vi "cryo v9.43.vi"() -> ()   [LabVIEW 2012]
uses:
  <vilib>/userdefined/High Color/IMAQdx.ctl
  <vilib>/Utility/file.llb/Read From Spreadsheet File (DBL).vi
  <vilib>/vision/driver/NI_Vision_Acquisition_Software.lvlib
  <vilib>/vision/NI_Vision_Development_Module.lvlib
panel:
  in  "Save\nImage":bool
  in  "Gap":u8=100
  in  "Position\nEstimate":dbl=20.0
  in  "Conn\nStm32":bool
  out "数值显示控件":dbl
  in  "停止按钮":bool
  in  "搜索按钮":bool
  out "Heater":u32(slide) scale=0.0..100.0
  out "数值 5":dbl
  out "数据显示 2":cluster{i32, dbl, dbl[][]}(graph)
  in  "文件路径输入控件 4":path=path "D:/testsizeout.txt"
  in  "多列列表框 3":i32(listbox)
  in  "Threshold Value":cluster{i32, i32}(slide)={180, 255} scale=0.0..255.0
  in  "文件路径输入控件 5":path=path "D:/testvideoin.avi"
  out "Source Image 5":T1(plugin-control) caption="Rejected Border"
  out "Source Image 4":T1(plugin-control) caption="Rejected Border"
  out "Source Image 3":T1(plugin-control) caption="Rejected Border"
  out "Source Image 2":T1(plugin-control) caption="Rejected Border"
  out "Source Image":T1(plugin-control) caption="Rejected Border"
  in  "Font, Size & Style":T2={"Desired Font (Application)"=enum."Application Font", "[User-specified Font]"={"Font Name"="", "Size"=12, "Strikeout?"=FALSE, "Italic?"=FALSE, "Underline?"=FALSE, "Outline?"=FALSE, "Shadow?"=FALSE, "Bold?"=FALSE, "Rotation Angle"=0.0}, "Horizontal Alignment"=0, "Vertical Alignment"=0} {"Vertical Alignment" items=["Bottom", "Top", "Baseline"]; "Horizontal Alignment" items=["Left", "Center", "Right"]; "[User-specified Font]"."Rotation Angle" format="%.2f"}
  in  "文件路径输入控件 3":path=path "D:/testvideoout.avi"
  in  "文件路径输入控件 2":path=path "D:/testprocessin.txt"
  in  "文件路径输入控件":path=path "D:/testtmpout.txt"
  in  "退出":bool
  in  "多列列表框 2":i32(listbox)
  in  "建立过程":bool
  in  "开始采集":bool
  out "数据显示":cluster{"x0":i32, "y":dbl, dbl[]}(graph)
  in  "停止采集":bool
  out "tmp":dbl(slide) scale=-50.0..50.0
  out "Injector 1":u32(slide) scale=0.0..100.0
  out "Injector 2":u32(slide) scale=0.0..100.0
  out "Injector 3":u32(slide) scale=0.0..100.0
  out "Refrigerator":u32(slide) scale=0.0..100.0
  out "数值 1":dbl
  out "数值 2":dbl
  out "数值 3":dbl
  out "数值 4":dbl
  out "多列列表框":i32[](listbox)
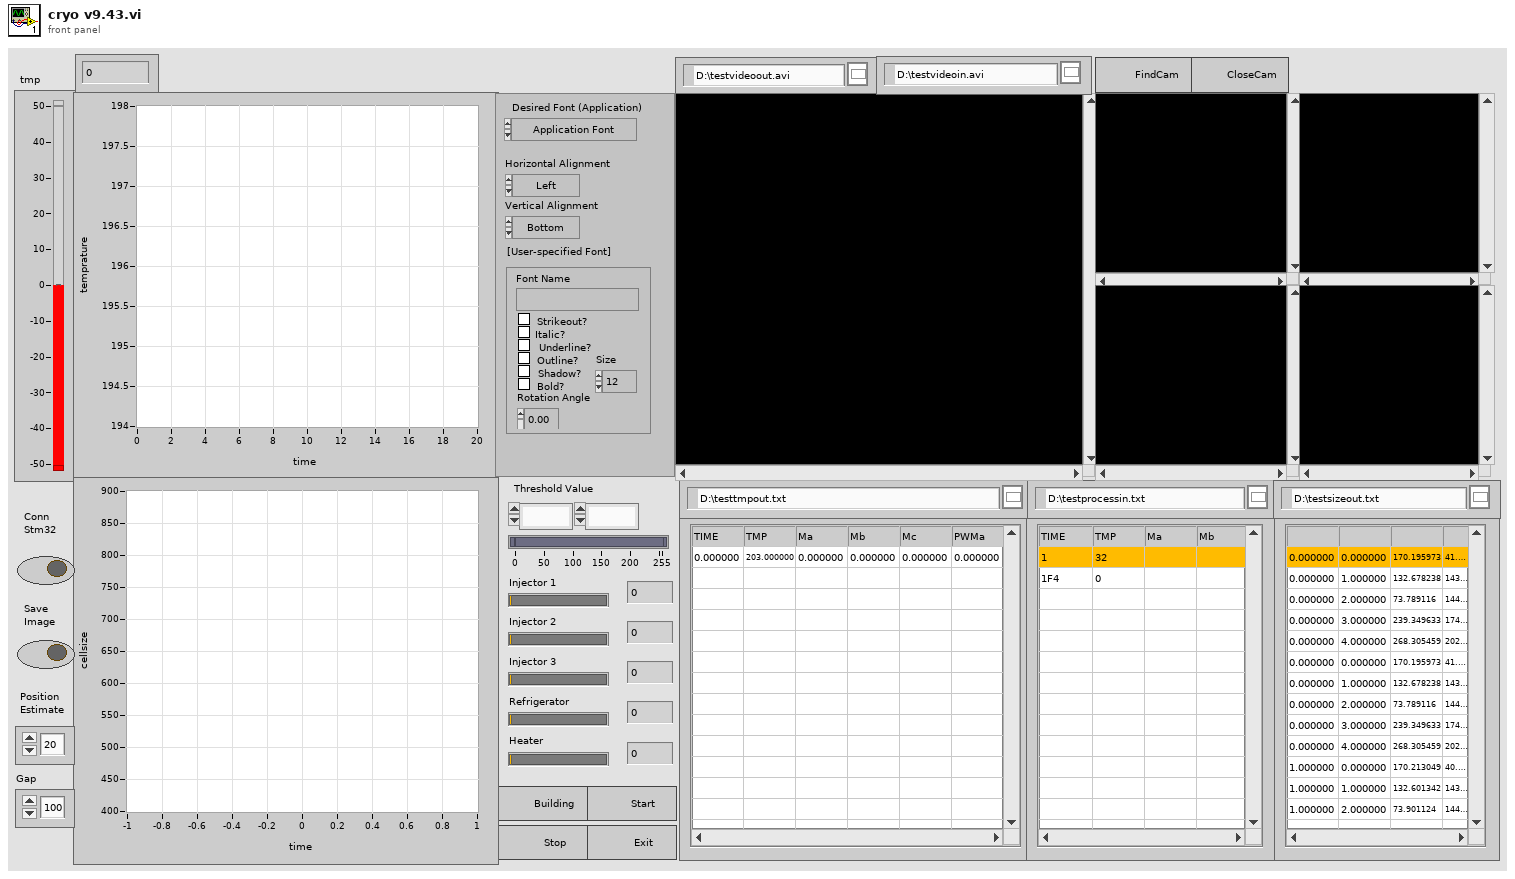
[diagram p1: front panel]
types:
  T1 = typedef "IMAQ Image.ctl" = refnum<image>
  T2 = cluster{"Desired Font (Application)":enum16{"User-specified Font", "Application Font", "System Font", "Dialog Font"}, "[User-specified Font]":cluster{"Font Name":string, "Size":i16, "Strikeout?":bool, "Italic?":bool, "Underline?":bool, "Outline?":bool, "Shadow?":bool, "Bold?":bool, "Rotation Angle":dbl}, "Horizontal Alignment":i16, "Vertical Alignment":i16}
  T3 = typedef "AviRefnum.ctl" = refnum<k1>
  T4 = typedef "Particle Parameters" = i32
  T5 = cluster{"Measurement Parameter":T4, "Range Lower Value":dbl, "Range Upper Value":dbl, "Range":bool, "Measurement Type":bool}[]
  T6 = enum32{"", "Gradient", "Laplacian", "Smoothing", "Gaussian"}
  T7 = cluster{"Particle Measurements (Pixels)[0]":dbl, "Particle Measurements (Pixels)[1]":dbl, "Particle Measurements (Pixels)[2]":dbl}
  T8 = cluster{"Particle Measurements (Pixels)[0]":dbl, "Particle Measurements (Pixels)[1]":dbl}
  T9 = cluster{i32, "Particle Measurements (Pixels)[0]":dbl, "Particle Measurements (Pixels)[1]":dbl, "Particle Measurements (Pixels)[2]":dbl, i32}
  T10 = cluster{i32, "Particle Measurements (Pixels)[0]":dbl, "Particle Measurements (Pixels)[1]":dbl, "Particle Measurements (Pixels)[2]":dbl, i32}[]
  T11 = typedef "IMAQdx.ctl" = refnum<k21>
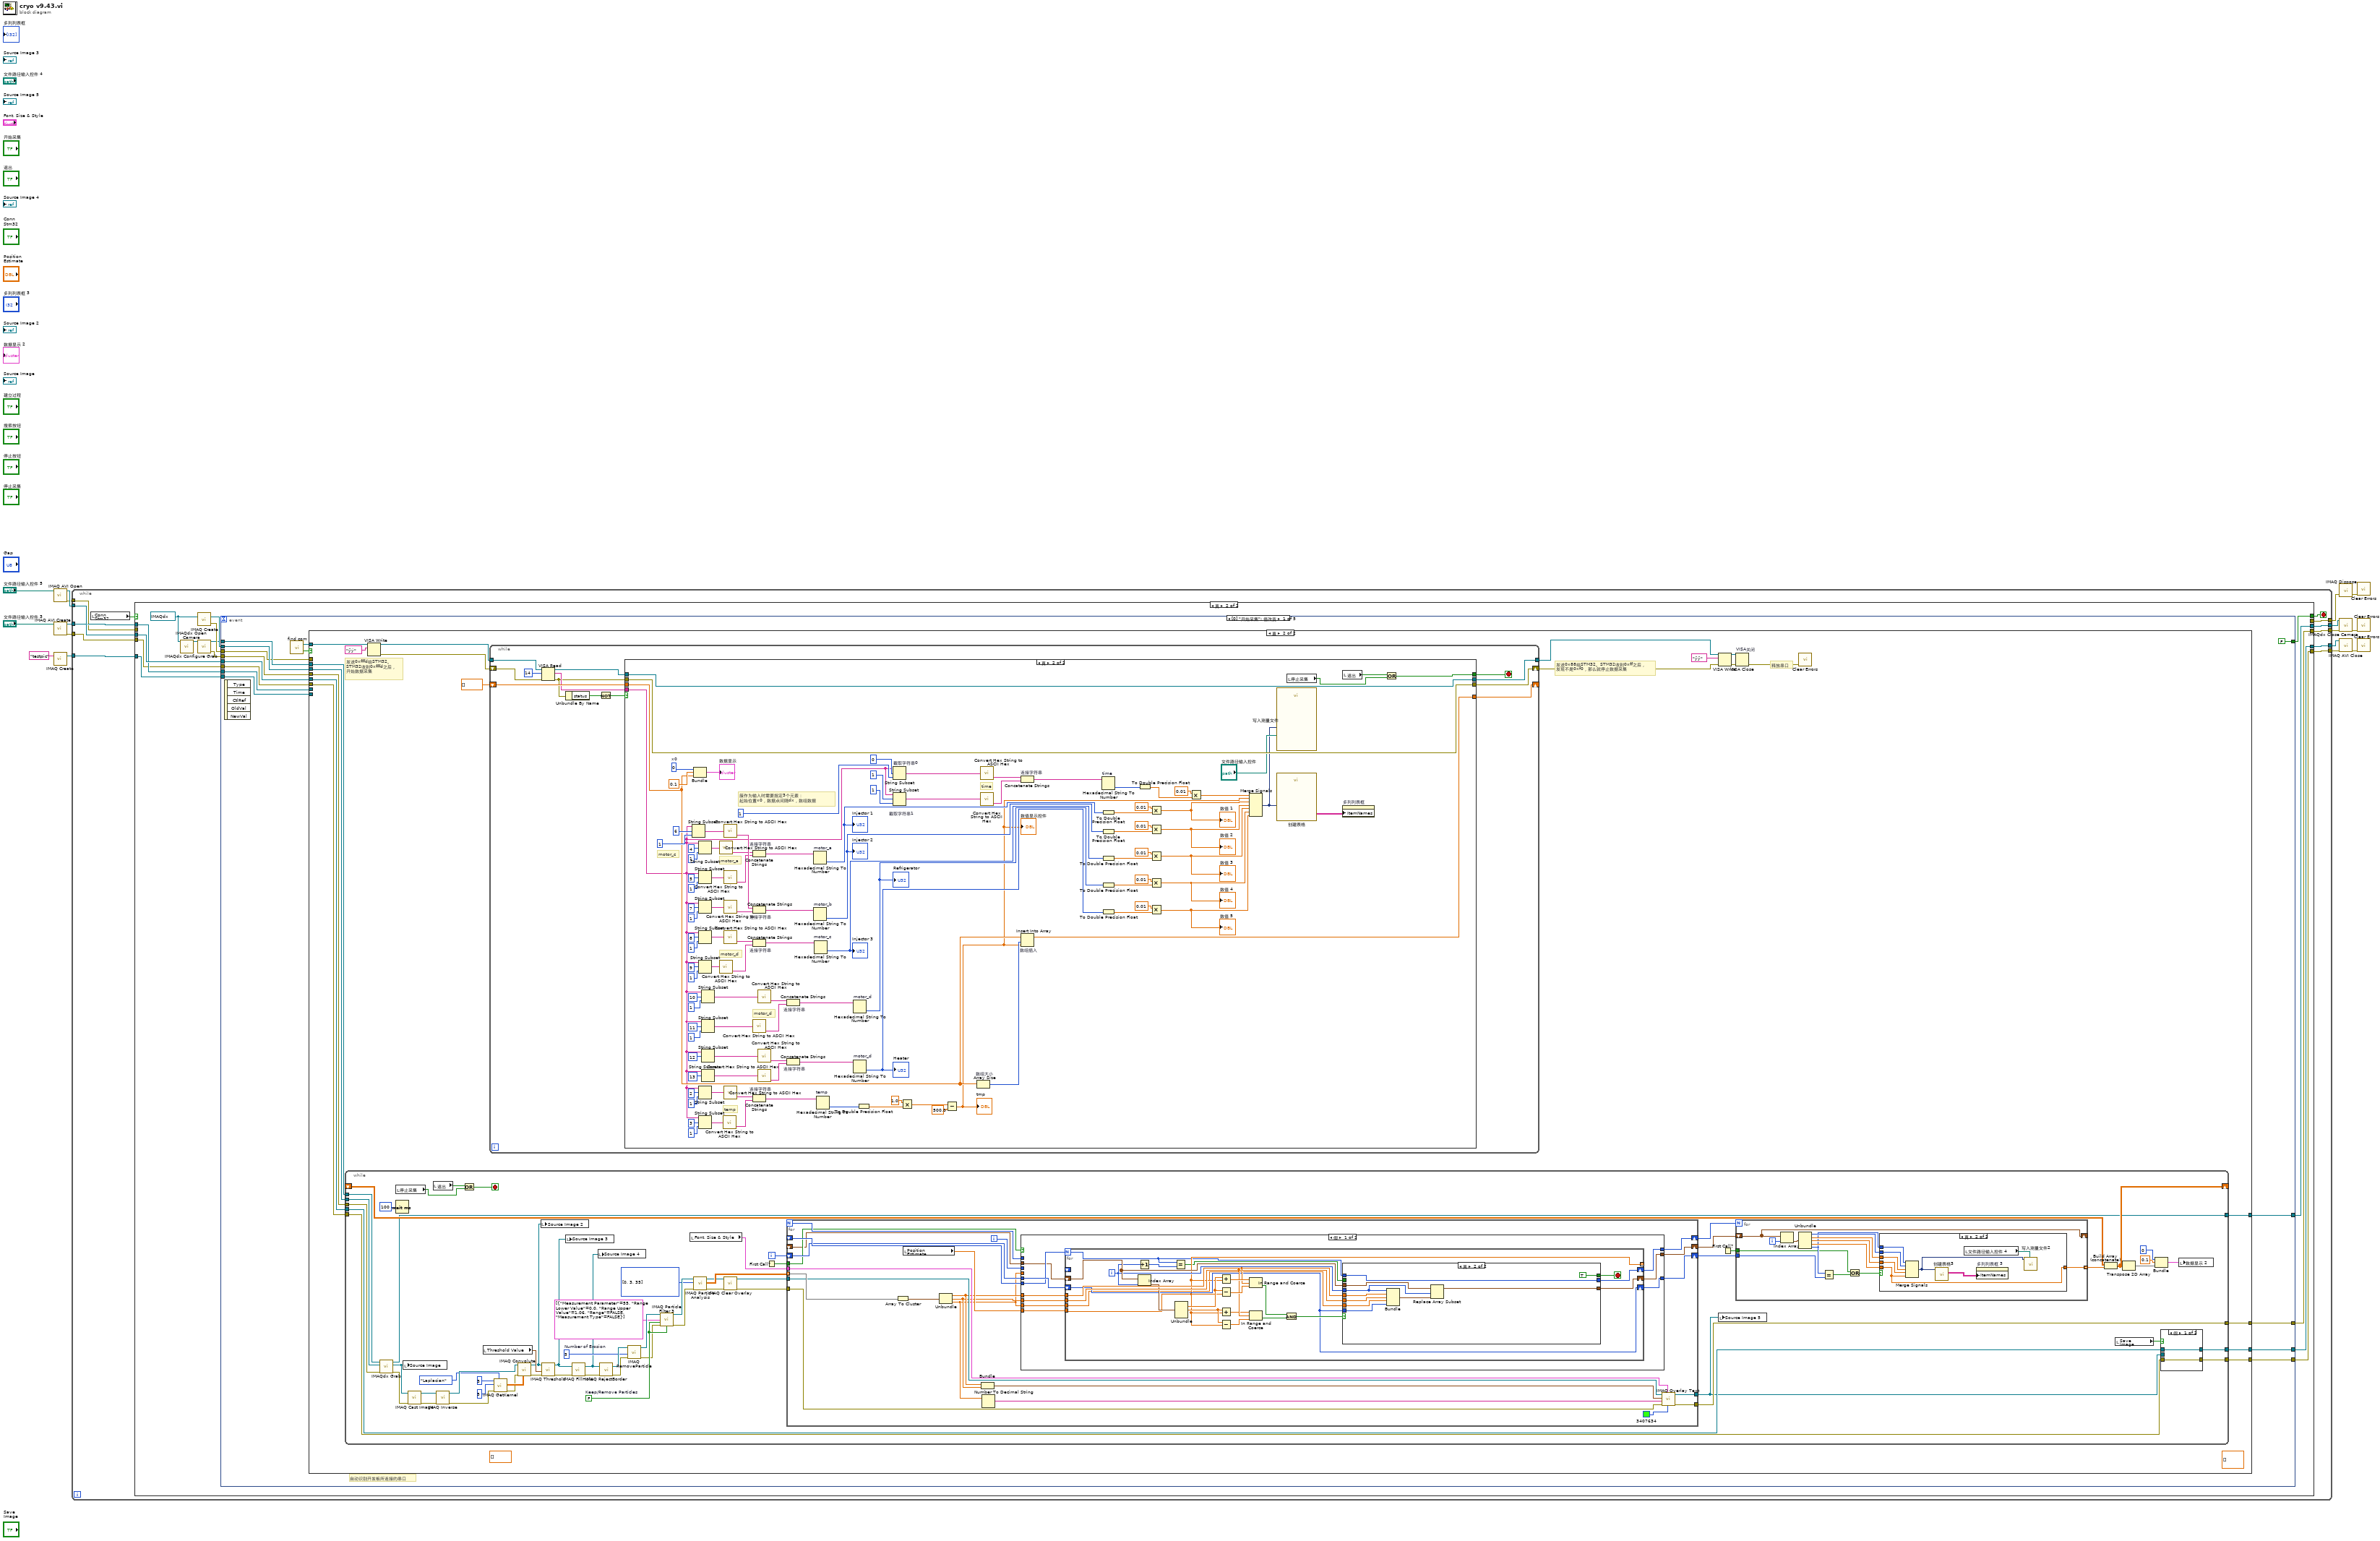
[diagram p0: block diagram]
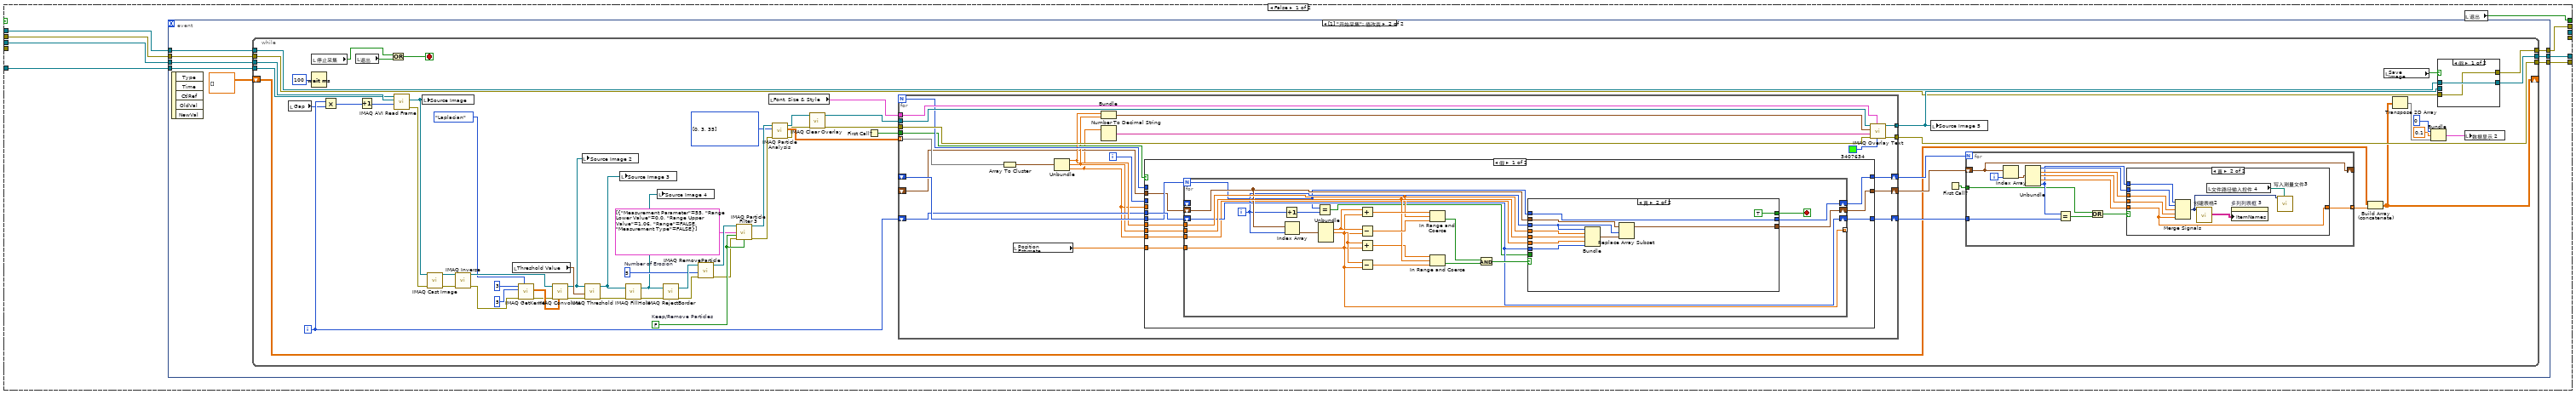
[diagram p2: hidden frame]
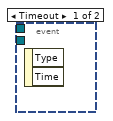
[diagram p3: hidden frame]
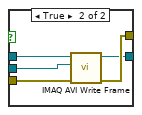
[diagram p4: hidden frame]
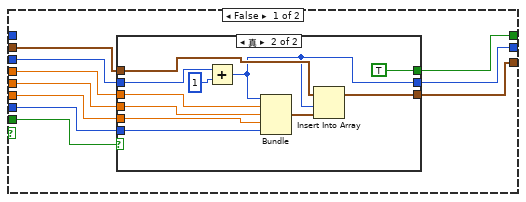
[diagram p6: hidden frame]
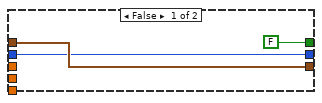
[diagram p7: hidden frame]
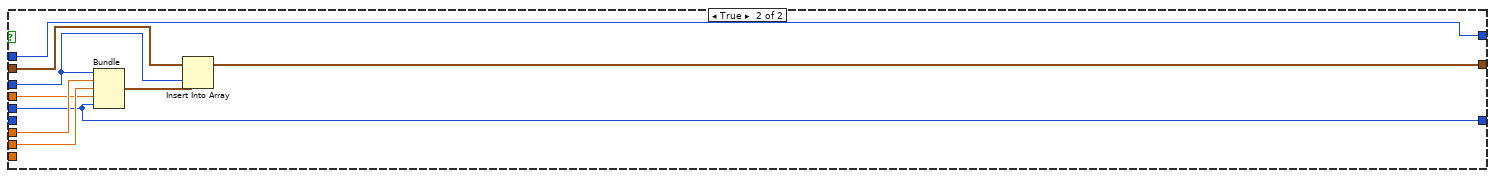
[diagram p8: hidden frame]
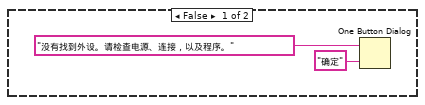
[diagram p9: hidden frame]
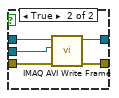
[diagram p10: hidden frame]
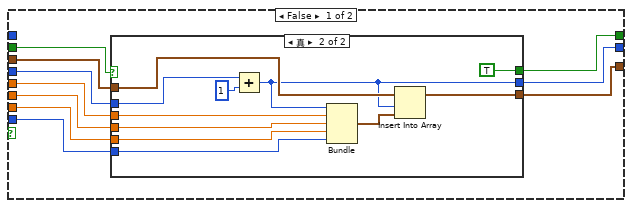
[diagram p12: hidden frame]
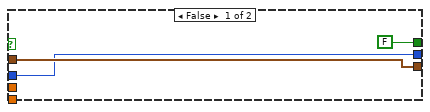
[diagram p13: hidden frame]
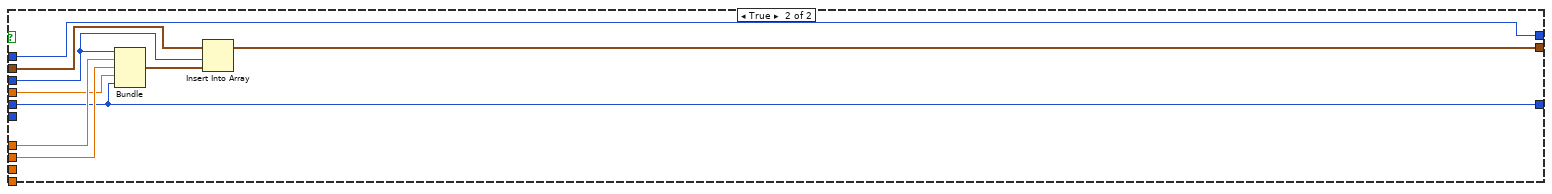
[diagram p14: hidden frame]
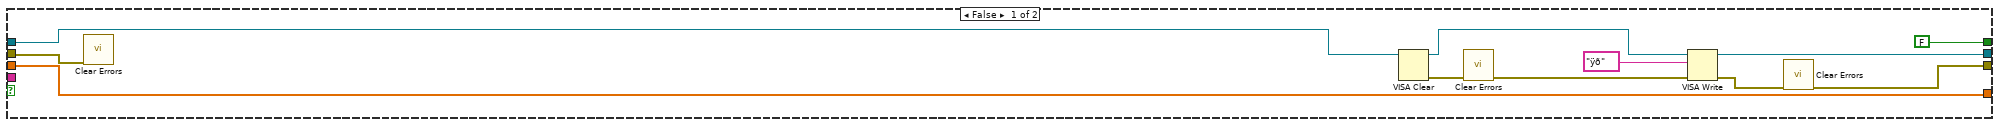
[diagram p15: hidden frame]
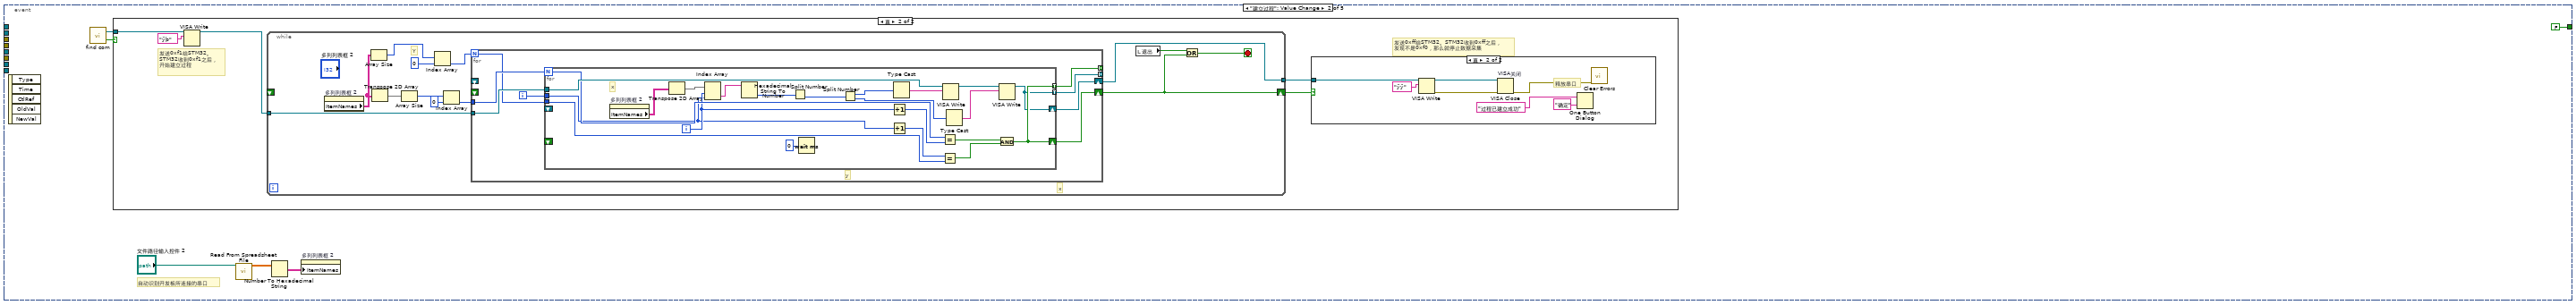
[diagram p16: hidden frame]
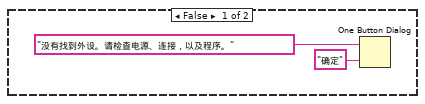
[diagram p17: hidden frame]
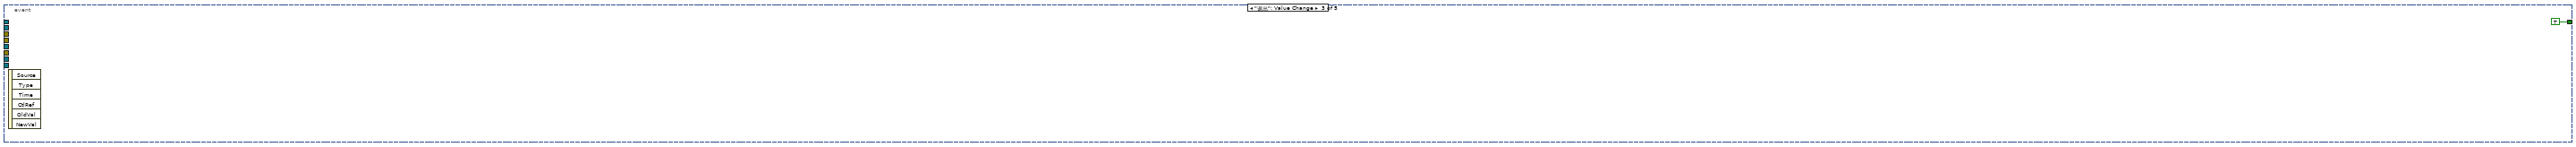
[diagram p19: hidden frame]
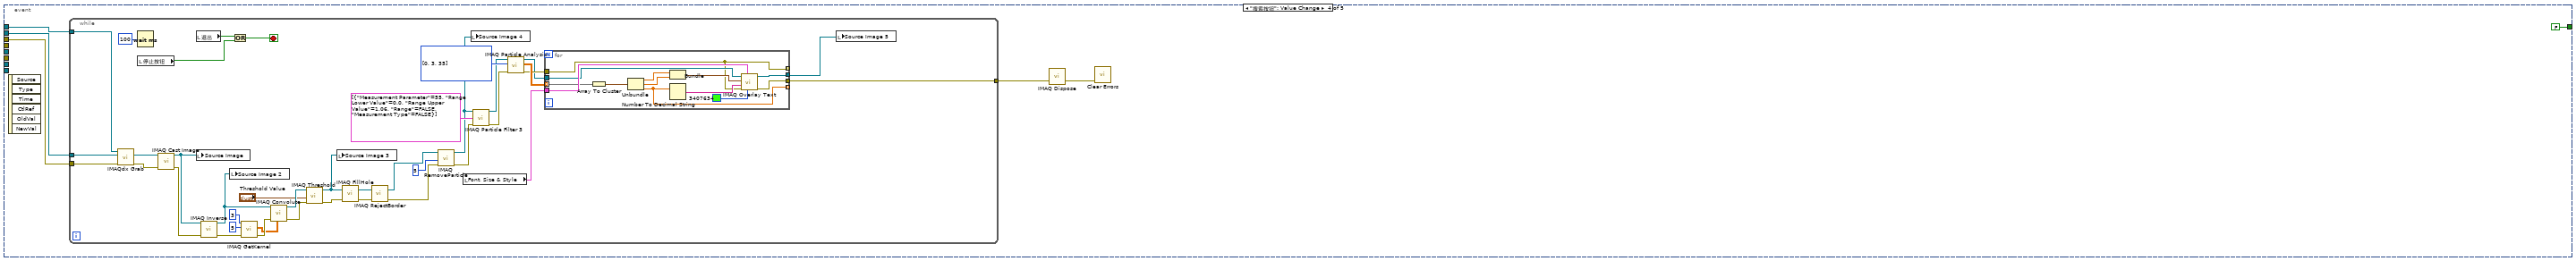
[diagram p20: hidden frame]
diagram:
  n1 = call "IMAQ AVI Open"("AVI Path"="文件路径输入控件 5") -> ("error out"=w4:errorcluster, "Avi Refnum"=w7:T3)  [unwired: 9 in]
  n2 = call "IMAQ AVI Create"("AVI Path"="文件路径输入控件 3") -> ("error out"=w1:errorcluster, "Avi Refnum"=w6:T3)  [unwired: 9 in]
  n3 = call "IMAQ Create"("Image Name"="testpic") -> ("New Image"=w8:T1)  [unwired: 4 in, 1 out]
  n4 = while {
    tunnel: [w27] -> w14
    tunnel: [w26] -> w12
    tunnel: [w28] -> w11
    tunnel: w8 -> [w24]
    tunnel: w7 -> [w23]
    tunnel: w6 -> [w22]
    tunnel: w4 -> [w20]
    tunnel: [w19] -> w3
    tunnel: [w18] -> w2
    tunnel: w1 -> [w17]
    stop <- w25 stop-if-true
    n5 = local read "Conn\nStm32"() -> (w21:bool)
    n6 = case shown="真" w21 {
      tunnel: [w32 _] -> w28
      tunnel: [w31 w236] -> w27
      tunnel: [w30 w240] -> w26
      tunnel: [w29 w250] -> w25
      tunnel: w24 -> [w36 w243]
      tunnel: w23 -> [w35 w242]
      tunnel: w22 -> [w33 w241]
      tunnel: w20 -> [w34 _]
      tunnel: [_ w239] -> w19
      tunnel: [_ w238] -> w18
      tunnel: w17 -> [_ w237]
      frame False {
        n7 = event shown="[1] \"开始采集\": 值改变" {
          selector: _ -> [_ _]
          dyn-events: _ -> [_ _]
          timeout: _ -> [_ _]
          tunnel: w36 -> [_ w43]
          tunnel: w35 -> [_ w42]
          tunnel: w34 -> [_ w41]
          tunnel: w33 -> [_ w40]
          tunnel: [_ w39] -> w32
          tunnel: [_ w38] -> w31
          tunnel: [_ w37] -> w30
          event Timeout {
            n8 = event-data() -> ()  [unwired: 1 in, 2 out]
          }
          event "开始采集": Value Change {
            n9 = event-data() -> ()  [unwired: 1 in, 5 out]
            n10 = while {
              tunnel: [w45] -> w38
              tunnel: w41 -> [w47]
              tunnel: w40 -> [w49]
              tunnel: [w46] -> w39
              tunnel: [w85] -> w37
              tunnel: w43 -> [w80]
              tunnel: w42 -> [w79]
              shift-right: [w58] -> _
              shift-left: dbl[][] [] -> [w59]
              i -> [w64]
              stop <- w82 stop-if-true
              w105 = T4[] [0, 3, 35] items=["Center of Mass X", "Center of Mass Y", "First Pixel X", "First Pixel Y", "Bounding Rect Left", "Bounding Rect Top", "Bounding Rect Right", "Bounding Rect Bottom", "Max Feret Diameter Start X", "Max Feret Diameter Start Y", "Max Feret Diameter End X", "Max Feret Diameter End Y", "Max Horiz. Segment Length Left", "Max Horiz. Segment Length Right", "Max Horiz. Segment Length Row", "-", "Bounding Rect Width", "Bounding Rect Height", "Bounding Rect Diagonal", "Perimeter", "Convex Hull Perimeter", "Holes' Perimeter", "Max Feret Diameter", "Equivalent Ellipse Major Axis", "Equivalent Ellipse Minor Axis", "Equivalent Ellipse Minor Axis (Feret)", "Equivalent Rect Long Side", "Equivalent Rect Short Side", "Equivalent Rect Diagonal", "Equivalent Rect Short Side (Feret)", "Average Horiz. Segment Length", "Average Vert. Segment Length", "Hydraulic Radius", "Waddel Disk Diameter", "-", "Area", "Holes' Area", "Particle & Holes' Area", "Convex Hull Area", "Image Area", "-", "Number of Holes", "Number of Horiz. Segments", "Number of Vert. Segments", "-", "Orientation", "Max Feret Diameter Orientation", "-", "% Area/Image Area", "% Area/(Particle & Holes' Area)", "Ratio of Equivalent Ellipse Axes", "Ratio of Equivalent Rect Sides", "-", "Elongation Factor", "Compactness Factor", "Heywood Circularity Factor", "Type Factor", "-", "Sum X", "Sum Y", "Sum XX", "Sum XY", "Sum YY", "Sum XXX", "Sum XXY", "Sum XYY", "Sum YYY", "-", "Moment of Inertia XX", "Moment of Inertia XY", "Moment of Inertia YY", "Moment of Inertia XXX", "Moment of Inertia XXY", "Moment of Inertia XYY", "Moment of Inertia YYY", "Norm. Moment of Inertia XX", "Norm. Moment of Inertia XY", "Norm. Moment of Inertia YY", "Norm. Moment of Inertia XXX", "Norm. Moment of Inertia XXY", "Norm. Moment of Inertia XYY", "Norm. Moment of Inertia YYY", "Hu Moment 1", "Hu Moment 2", "Hu Moment 3", "Hu Moment 4", "Hu Moment 5", "Hu Moment 6", "Hu Moment 7"] ("Pixel Measurements")
              w93 = 5  # Number of Erosion
              w95 = FALSE  # Keep/Remove Particles
              n11 = local read "Gap"() -> (w51:u8)
              n12 = local read "停止采集"() -> (w84:bool)
              n13 = Wait (ms)(milliseconds to wait=100) -> ()  [unwired: 1 out]
              n14 = Multiply(x=w64, y=w51) -> (x*y=w54:i32)
              n15 = local read "退出"() -> (w83:bool)
              n16 = Increment(x=w54) -> (x+1=w53:i32)
              n17 = Or(x=w84, y=w83) -> (x .or. y?=w82:bool)
              n18 = call "IMAQ AVI Read Frame"("Frame Number"=w53, "Image"=w80, "Avi Refnum"=w79) -> ("error out"=w52:errorcluster, "Image Out"=w68:T1)  [unwired: 5 in, 2 out]
              n19 = local write "Source Image"(w68) -> ()
              n20 = call "IMAQ Cast Image"("error in (no error)"=w52, "Image Src"=w68) -> ("error out"=w102:errorcluster, "Image Dst Out"=w81:T1)  [unwired: 8 in]
              n21 = call "IMAQ Inverse"("error in (no error)"=w102, "Image Src"=w81) -> ("error out"=w101:errorcluster, "Image Dst Out"=w91:T1)  [unwired: 8 in]
              n22 = local read "Threshold Value"() -> (w71:cluster{i32, i32})
              n23 = call "IMAQ GetKernel"("Kernel Family"=T6."Laplacian", "error in (no error)"=w101, "Kernel Number"=5, "Kernel Size (3,5,...)"=3) -> ("error out"=w86:errorcluster, "Kernel"=w87:sgl[][])  [unwired: 1 in, 5 out]
              n24 = call "IMAQ Convolute"("Kernel"=w87, "error in (no error)"=w86, "Image Src"=w91) -> ("error out"=w100:errorcluster, "Image Dst Out"=w67:T1)  [unwired: 4 in, 3 out]
              n25 = local write "Source Image 2"(w67) -> ()
              n26 = call "IMAQ Threshold"("error in (no error)"=w100, "Range"=w71, "Image Src"=w67) -> ("error out"=w97:errorcluster, "Image Dst Out"=w66:T1)  [unwired: 3 in, 4 out]
              n27 = local write "Source Image 3"(w66) -> ()
              n28 = call "IMAQ FillHole"("error in (no error)"=w97, "Image Src"=w66) -> ("error out"=w98:errorcluster, "Image Dst Out"=w65:T1)  [unwired: 2 in, 2 out]
              n29 = local write "Source Image 4"(w65) -> ()
              n30 = call "IMAQ RejectBorder"("error in (no error)"=w98, "Image Src"=w65) -> ("error out"=w99:errorcluster, "Image Dst Out"=w96:T1)  [unwired: 2 in, 2 out]
              n31 = call "IMAQ RemoveParticle"("error in (no error)"=w99, "Number of Erosion"=w93, "Image Src"=w96) -> ("error out"=w92:errorcluster, "Image Dst Out"=w103:T1)  [unwired: 4 in, 3 out]
              n32 = call "IMAQ Particle Filter 3"("Image Src"=w103, "Selection Values"=T5 [{"Measurement Parameter"=55, "Range Lower Value"=0.0, "Range Upper Value"=1.06, "Range"=FALSE, "Measurement Type"=FALSE}], "Keep/Remove Particles (F)"=w95, "error in (no error)"=w92, "Fill Holes? (F)"=w95) -> ("Image Dst Out"=w106:T1, "error out"=w107:errorcluster)  [unwired: 4 in, 5 out]
              n33 = local read "Font, Size & Style"() -> (w69:T2)
              n34 = call "IMAQ Particle Analysis"("error in (no error)"=w107, "Pixel Measurements"=w105, "Image"=w106) -> ("error out"=w76:errorcluster, "Particle Measurements (Pixels)"=w104:dbl[][], "Image Out (duplicate)"=w78:T1)  [unwired: 2 in, 4 out]
              n35 = call "IMAQ Clear Overlay"("error in (no error)"=w76, "Image"=w78) -> ("error out"=w75:errorcluster, "Image Out"=w77:T1)  [unwired: 8 in]
              n36 = First Call?() -> (First Call?: T/F=w56:bool)
              n37 = for "For循环" {
                N -> [w149]
                tunnel: w75 -> [w159]
                tunnel: [w158] -> w85
                tunnel: [w157] -> w48
                tunnel: w69 -> [w152]
                tunnel: w104 -> [w151] mode=indexing
                tunnel: w77 -> [w150]
                shift-right: [w143] -> w62
                shift-left: _ -> [w148]
                shift-right: [w144] -> w61
                shift-left: w64 -> [w145]
                shift-right: [w142] -> w63
                shift-left: _ -> [w138]
                tunnel: w56 -> [w141]
                i -> [w140]
                n38 = Array To Cluster(array=w151) -> (cluster=w154:T7)
                n39 = local read "Position\nEstimate"() -> (w147:dbl)
                n40 = Unbundle(w154) -> ("Particle Measurements (Pixels)[0]"=w146:dbl, "Particle Measurements (Pixels)[1]"=w139:dbl, "Particle Measurements (Pixels)[2]"=w137:dbl)
                n41 = Bundle("Particle Measurements (Pixels)[0]"=w146, "Particle Measurements (Pixels)[1]"=w139) -> (w153:T8)  [unwired: 1 out]
                n42 = Number To Decimal String(number=w137) -> (decimal integer string=w156:string)  [unwired: 1 out]
                n43 = case shown="假" w141 {
                  tunnel: w149 -> [_ w232]
                  tunnel: w148 -> [w162 _]
                  tunnel: w147 -> [w169 _]
                  tunnel: w146 -> [w168 w235]
                  tunnel: w137 -> [w167 _]
                  tunnel: w145 -> [w166 w231]
                  tunnel: [w165 w231] -> w144
                  tunnel: [w160 w232] -> w143
                  tunnel: [w164 w229] -> w142
                  tunnel: w140 -> [_ w227]
                  tunnel: w139 -> [w163 w234]
                  tunnel: w137 -> [_ w233]
                  tunnel: w138 -> [w161 w230]
                  frame False {
                    n44 = for {
                      N: w162 -> [w171]
                      tunnel: w168 -> [w186]
                      tunnel: [w176] -> _ mode=indexing
                      tunnel: w163 -> [w187]
                      tunnel: w167 -> [w174]
                      shift-right: [w173] -> w164
                      shift-left: w161 -> [w185]
                      shift-right: [w172] -> w160
                      shift-left: _ -> [_]
                      shift-right: [w179] -> w165
                      shift-left: w166 -> [w179]
                      tunnel: w169 -> [w176]
                      i -> [w178]
                      stop <- w170 stop-if-true
                      n45 = Increment(x=w178) -> (x+1=w177:i32)
                      n46 = Index Array(array=w185, index=w178) -> (element=w184:T9)
                      n47 = Equal?(x=w171, y=w177) -> (x = y?=w175:bool)
                      n48 = Unbundle(w184) -> ("Particle Measurements (Pixels)[0]"=w183:dbl, "Particle Measurements (Pixels)[1]"=w182:dbl)  [unwired: 3 out]
                      n49 = Add(x=w183, y=w176) -> (x+y=w192:dbl)
                      n50 = Subtract(x=w183, y=w176) -> (x-y=w191:dbl)
                      n51 = Add(x=w182, y=w176) -> (x+y=w181:dbl)
                      n52 = Subtract(x=w182, y=w176) -> (x-y=w180:dbl)
                      n53 = In Range and Coerce(upper limit=w192, x=w186, lower limit=w191) -> (In Range?=w190:bool)  [unwired: 1 out]
                      n54 = In Range and Coerce(upper limit=w181, x=w187, lower limit=w180) -> (In Range?=w189:bool)  [unwired: 1 out]
                      n55 = And(x=w190, y=w189) -> (x .and. y?=w188:bool)
                      n56 = case shown="真" w188 {
                        tunnel: w178 -> [w198 w220]
                        tunnel: w186 -> [w197 w226]
                        tunnel: w187 -> [w194 w225]
                        tunnel: w174 -> [w199 w224]
                        tunnel: w185 -> [w201 w223]
                        tunnel: [w200 w222] -> w173
                        tunnel: w179 -> [w196 w219]
                        tunnel: w175 -> [w202 _]
                        tunnel: [w195 w218] -> w172
                        tunnel: w171 -> [_ w218]
                        tunnel: [w193 TRUE] -> w170
                        frame False {
                          n57 = case shown="真" w202 {
                            tunnel: w201 -> [w205 w216]
                            tunnel: [w205 w215] -> w200
                            tunnel: w194 -> [_ w207]
                            tunnel: w197 -> [_ w214]
                            tunnel: w198 -> [w204 w213]
                            tunnel: [w204 w211] -> w195
                            tunnel: w196 -> [_ w210]
                            tunnel: w199 -> [_ w208]
                            tunnel: [FALSE TRUE] -> w193
                            frame False {
                            }
                            frame True {
                              n58 = Add(x=w213, y=1) -> (x+y=w211:i32)
                              n59 = Bundle(w211, "Particle Measurements (Pixels)[0]"=w214, "Particle Measurements (Pixels)[1]"=w207, "Particle Measurements (Pixels)[2]"=w208, w210) -> (w209:T9)  [unwired: 1 out]
                              n60 = Insert Into Array(array=w216, index=w211, new element=w209) -> (w215:T10)
                            }
                          }
                        }
                        frame True {
                          n61 = Bundle(w220, "Particle Measurements (Pixels)[0]"=w226, "Particle Measurements (Pixels)[1]"=w225, "Particle Measurements (Pixels)[2]"=w224, w219) -> (w221:T9)  [unwired: 1 out]
                          n62 = Replace Array Subset(array=w223, new element=w221, index=w220) -> (w222:T10)
                        }
                      }
                    }
                  }
                  frame True {
                    n63 = Bundle(w227, "Particle Measurements (Pixels)[0]"=w235, "Particle Measurements (Pixels)[1]"=w234, "Particle Measurements (Pixels)[2]"=w233, w231) -> (w228:T9)  [unwired: 1 out]
                    n64 = Insert Into Array(array=w230, index=w227, new element=w228) -> (w229:T10)
                  }
                }
                n65 = call "IMAQ Overlay Text"("Text Color (black)"=u32 3407634, "Font, Size & Style"=w152, "error in (no error)"=w159, "String"=w156, "Origin"=w153, "Image"=w150) -> ("error out"=w158:errorcluster, "Image Out"=w157:T1)  [unwired: 2 in, 2 out]
              }
              n66 = local write "Source Image 5"(w48) -> ()
              n67 = First Call?() -> (First Call?: T/F=w55:bool)
              n68 = for {
                N: w62 -> [_]
                shift-right: [w118] -> _
                shift-left: w63 -> [w118]
                tunnel: w61 -> [w121]
                tunnel: [w119] -> w60 mode=indexing
                tunnel: w55 -> [w116]
                i -> [w127]
                n69 = Index Array(array=w118, index=w127) -> (element=w126:T9)
                n70 = Unbundle(w126) -> (w125:i32, "Particle Measurements (Pixels)[0]"=w124:dbl, "Particle Measurements (Pixels)[1]"=w123:dbl, "Particle Measurements (Pixels)[2]"=w122:dbl, w120:i32)
                n71 = Equal?(x=w120, y=w121) -> (x = y?=w117:bool)
                n72 = Or(x=w116, y=w117) -> (x .or. y?=w115:bool)
                n73 = case shown="真" w115 {
                  tunnel: w125 -> [_ w131]
                  tunnel: w124 -> [_ w133]
                  tunnel: w123 -> [_ w132]
                  tunnel: w122 -> [w128 w129]
                  tunnel: w120 -> [_ w130]
                  tunnel: [w128 w129] -> w119
                  frame False {
                  }
                  frame True {
                    n74 = Merge Signals(w130, w131, w133, w132, w129) -> (w134:dynamicdata)
                    n75 = call "创建表格2"("Signals"=w134) -> ("Table"=w135:string[][])  [unwired: 9 in, 1 out]
                    n76 = local read "文件路径输入控件 4"() -> (w136:path)
                    n77 = property on="多列列表框 3" class="MCListbox (严格)"("ItemNames"=w135) -> ()  [unwired: 2 in, 2 out]
                    n78 = call "写入测量文件3"("Signals"=w134, "Filename"=w136) -> ()  [unwired: 15 in, 3 out]
                  }
                }
              }
              n79 = Build Array (concatenate)(w59, w60) -> (w58:dbl[][])
              n80 = local read "Save\nImage"() -> (w50:bool)
              n81 = Transpose 2D Array(2D array=w58) -> (transposed array=w72:dbl[][])
              n82 = Bundle(0, 0.1, w72) -> (w70:cluster{i32, dbl, dbl[][]})  [unwired: 1 out]
              n83 = case shown="假" w50 {
                tunnel: w49 -> [w109 w114]
                tunnel: w48 -> [_ w113]
                tunnel: w47 -> [w108 w112]
                tunnel: [w108 w111] -> w46
                tunnel: [w109 w110] -> w45
                frame False {
                }
                frame True {
                  n84 = call "IMAQ AVI Write Frame"("error in (no error)"=w112, "Image"=w113, "Avi Refnum"=w114) -> ("error out"=w111:errorcluster, "Avi Refnum (duplicate)"=w110:T3)  [unwired: 7 in]
                }
              }
              n85 = local write "数据显示 2"(w70) -> ()
            }
          }
        }
        n86 = local read "退出"() -> (w29:bool)
      }
      frame True {
        w249 = T11 "cam0" ("Session In")
        n87 = call <vilib>:"IMAQdx Open Camera.vi"("Session In"=w249) -> ("Session Out"=w248:T11)  [unwired: 9 in, 1 out]
        n88 = call "IMAQ Create"("Image Name"=w249) -> ("New Image"=w246:T1, "error out"=w247:errorcluster)  [unwired: 4 in]
        n89 = call <vilib>:"IMAQdx Configure Grab.vi"("Session In"=w248) -> ("error out"=w245:errorcluster, "Session Out"=w244:T11)  [unwired: 1 in, 8 out]
        n90 = event shown="[0] \"开始采集\": 值改变" {
          selector: _ -> [_ _ _ _ _]
          dyn-events: _ -> [_ _ _ _ _]
          timeout: _ -> [_ _ _ _ _]
          tunnel: [FALSE ("停止采集") FALSE ("保存按钮") TRUE ("停止采集") FALSE FALSE ("停止采集")] -> w250
          tunnel: w241 -> [w262 _ _ _ _]
          tunnel: w246 -> [w261 _ _ w674 _]
          tunnel: w244 -> [w260 _ _ w673 _]
          tunnel: w247 -> [w259 _ _ w675 _]
          tunnel: w245 -> [w258 _ _ _ _]
          tunnel: w243 -> [w257 _ _ _ _]
          tunnel: w242 -> [w256 _ _ _ _]
          tunnel: [w255 _ _ _ _] -> w240
          tunnel: [w254 _ _ _ _] -> w239
          tunnel: [w253 _ _ _ _] -> w238
          tunnel: w237 -> [w252 _ _ _ _]
          tunnel: [w251 _ _ _ _] -> w236
          event "开始采集": Value Change {
            # "自动识别开发板所连接的串口"
            n91 = event-data() -> ()  [unwired: 6 out]
            n92 = call "find com.vi"() -> ("连接了开发板？"=w264:bool, "VISA resource name out"=w265:refnum<visa-resource-name>)  [unwired: 2 in]
            n93 = case shown="真" w264 {
              tunnel: w265 -> [_ w280]
              tunnel: w262 -> [_ _]
              tunnel: w261 -> [_ w274]
              tunnel: w260 -> [_ w276]
              tunnel: w259 -> [_ _]
              tunnel: w258 -> [_ w275]
              tunnel: w257 -> [_ _]
              tunnel: w256 -> [_ w271]
              tunnel: [_ w273] -> w255
              tunnel: [_ w272] -> w254
              tunnel: [_ w270] -> w253
              tunnel: w252 -> [_ w269]
              tunnel: [_ w268] -> w251
              frame False {
                n94 = One Button Dialog(message="没有找到外设。请检查电源、连接，以及程序。" ("消息"), button name ("OK")="确定" ("按钮名称（“确定”）")) -> ()  [unwired: 1 out]
              }
              frame True {
                (unwired) dbl[] []
                (unwired) dbl[][] []
                # "发送0x88给STM32。STM32收到0xff之后，\n发现不是0xf0，那么就停止数据采集"
                # "发送0xfffd给STM32。\nSTM32收到0xfffd之后，\n开始数据采集"
                # "释放串口"
                n95 = while {
                  tunnel: [w289] -> w273
                  tunnel: [w327] -> w272
                  shift-right: [w303] -> _
                  shift-left: _ -> [w304]
                  tunnel: w276 -> [w297]
                  tunnel: w275 -> [w296]
                  tunnel: w274 -> [w295]
                  tunnel: w271 -> [w292]
                  tunnel: [w294] -> w270
                  tunnel: w269 -> [w290]
                  tunnel: [w288] -> w268
                  i -> [w309]
                  stop <- w324 stop-if-true
                  w347 = T4[] [0, 3, 35] items=["Center of Mass X", "Center of Mass Y", "First Pixel X", "First Pixel Y", "Bounding Rect Left", "Bounding Rect Top", "Bounding Rect Right", "Bounding Rect Bottom", "Max Feret Diameter Start X", "Max Feret Diameter Start Y", "Max Feret Diameter End X", "Max Feret Diameter End Y", "Max Horiz. Segment Length Left", "Max Horiz. Segment Length Right", "Max Horiz. Segment Length Row", "-", "Bounding Rect Width", "Bounding Rect Height", "Bounding Rect Diagonal", "Perimeter", "Convex Hull Perimeter", "Holes' Perimeter", "Max Feret Diameter", "Equivalent Ellipse Major Axis", "Equivalent Ellipse Minor Axis", "Equivalent Ellipse Minor Axis (Feret)", "Equivalent Rect Long Side", "Equivalent Rect Short Side", "Equivalent Rect Diagonal", "Equivalent Rect Short Side (Feret)", "Average Horiz. Segment Length", "Average Vert. Segment Length", "Hydraulic Radius", "Waddel Disk Diameter", "-", "Area", "Holes' Area", "Particle & Holes' Area", "Convex Hull Area", "Image Area", "-", "Number of Holes", "Number of Horiz. Segments", "Number of Vert. Segments", "-", "Orientation", "Max Feret Diameter Orientation", "-", "% Area/Image Area", "% Area/(Particle & Holes' Area)", "Ratio of Equivalent Ellipse Axes", "Ratio of Equivalent Rect Sides", "-", "Elongation Factor", "Compactness Factor", "Heywood Circularity Factor", "Type Factor", "-", "Sum X", "Sum Y", "Sum XX", "Sum XY", "Sum YY", "Sum XXX", "Sum XXY", "Sum XYY", "Sum YYY", "-", "Moment of Inertia XX", "Moment of Inertia XY", "Moment of Inertia YY", "Moment of Inertia XXX", "Moment of Inertia XXY", "Moment of Inertia XYY", "Moment of Inertia YYY", "Norm. Moment of Inertia XX", "Norm. Moment of Inertia XY", "Norm. Moment of Inertia YY", "Norm. Moment of Inertia XXX", "Norm. Moment of Inertia XXY", "Norm. Moment of Inertia XYY", "Norm. Moment of Inertia YYY", "Hu Moment 1", "Hu Moment 2", "Hu Moment 3", "Hu Moment 4", "Hu Moment 5", "Hu Moment 6", "Hu Moment 7"] ("Pixel Measurements")
                  w335 = 5  # Number of Erosion
                  w337 = FALSE  # Keep/Remove Particles
                  n96 = call <vilib>:"IMAQdx Grab.vi"("error in"=w296, "Image In"=w295, "Session In"=w297) -> ("error out"=w298:errorcluster, "Image Out"=w299:T1, "Session Out"=w294:T11)  [unwired: 5 in, 1 out]
                  n97 = local read "停止采集"() -> (w325:bool)
                  n98 = Wait (ms)(milliseconds to wait=100) -> ()  [unwired: 1 out]
                  n99 = local write "Source Image"(w299) -> ()
                  n100 = call "IMAQ Cast Image"("error in (no error)"=w298, "Image Src"=w299) -> ("error out"=w344:errorcluster, "Image Dst Out"=w323:T1)  [unwired: 8 in]
                  n101 = local read "退出"() -> (w326:bool)
                  n102 = call "IMAQ Inverse"("error in (no error)"=w344, "Image Src"=w323) -> ("error out"=w343:errorcluster, "Image Dst Out"=w333:T1)  [unwired: 8 in]
                  n103 = Or(x=w326, y=w325) -> (x .or. y?=w324:bool)
                  n104 = local read "Threshold Value"() -> (w315:cluster{i32, i32})
                  n105 = call "IMAQ GetKernel"("Kernel Family"=T6."Laplacian", "error in (no error)"=w343, "Kernel Number"=5, "Kernel Size (3,5,...)"=3) -> ("error out"=w328:errorcluster, "Kernel"=w329:sgl[][])  [unwired: 1 in, 5 out]
                  n106 = call "IMAQ Convolute"("Kernel"=w329, "error in (no error)"=w328, "Image Src"=w333) -> ("error out"=w342:errorcluster, "Image Dst Out"=w312:T1)  [unwired: 4 in, 3 out]
                  n107 = local write "Source Image 2"(w312) -> ()
                  n108 = call "IMAQ Threshold"("error in (no error)"=w342, "Range"=w315, "Image Src"=w312) -> ("error out"=w339:errorcluster, "Image Dst Out"=w311:T1)  [unwired: 3 in, 4 out]
                  n109 = local write "Source Image 3"(w311) -> ()
                  n110 = call "IMAQ FillHole"("error in (no error)"=w339, "Image Src"=w311) -> ("error out"=w340:errorcluster, "Image Dst Out"=w310:T1)  [unwired: 2 in, 2 out]
                  n111 = local write "Source Image 4"(w310) -> ()
                  n112 = call "IMAQ RejectBorder"("error in (no error)"=w340, "Image Src"=w310) -> ("error out"=w341:errorcluster, "Image Dst Out"=w338:T1)  [unwired: 2 in, 2 out]
                  n113 = call "IMAQ RemoveParticle"("error in (no error)"=w341, "Number of Erosion"=w335, "Image Src"=w338) -> ("error out"=w334:errorcluster, "Image Dst Out"=w345:T1)  [unwired: 4 in, 3 out]
                  n114 = call "IMAQ Particle Filter 3"("Image Src"=w345, "Selection Values"=T5 [{"Measurement Parameter"=55, "Range Lower Value"=0.0, "Range Upper Value"=1.06, "Range"=FALSE, "Measurement Type"=FALSE}], "Keep/Remove Particles (F)"=w337, "error in (no error)"=w334, "Fill Holes? (F)"=w337) -> ("Image Dst Out"=w348:T1, "error out"=w349:errorcluster)  [unwired: 4 in, 5 out]
                  n115 = local read "Font, Size & Style"() -> (w313:T2)
                  n116 = call "IMAQ Particle Analysis"("error in (no error)"=w349, "Pixel Measurements"=w347, "Image"=w348) -> ("error out"=w320:errorcluster, "Particle Measurements (Pixels)"=w346:dbl[][], "Image Out (duplicate)"=w322:T1)  [unwired: 2 in, 4 out]
                  n117 = call "IMAQ Clear Overlay"("error in (no error)"=w320, "Image"=w322) -> ("error out"=w319:errorcluster, "Image Out"=w321:T1)  [unwired: 8 in]
                  n118 = First Call?() -> (First Call?: T/F=w301:bool)
                  n119 = for "For循环" {
                    N -> [w391]
                    tunnel: w319 -> [w401]
                    tunnel: [w400] -> w327
                    tunnel: [w399] -> w291
                    tunnel: w313 -> [w394]
                    tunnel: w346 -> [w393] mode=indexing
                    tunnel: w321 -> [w392]
                    shift-right: [w385] -> w307
                    shift-left: _ -> [w390]
                    shift-right: [w386] -> w306
                    shift-left: w309 -> [w387]
                    shift-right: [w384] -> w308
                    shift-left: _ -> [w380]
                    tunnel: w301 -> [w383]
                    i -> [w382]
                    n120 = Array To Cluster(array=w393) -> (cluster=w396:T7)
                    n121 = local read "Position\nEstimate"() -> (w389:dbl)
                    n122 = Unbundle(w396) -> ("Particle Measurements (Pixels)[0]"=w388:dbl, "Particle Measurements (Pixels)[1]"=w381:dbl, "Particle Measurements (Pixels)[2]"=w379:dbl)
                    n123 = Bundle("Particle Measurements (Pixels)[0]"=w388, "Particle Measurements (Pixels)[1]"=w381) -> (w395:T8)  [unwired: 1 out]
                    n124 = Number To Decimal String(number=w379) -> (decimal integer string=w398:string)  [unwired: 1 out]
                    n125 = case shown="假" w383 {
                      tunnel: w391 -> [_ w474]
                      tunnel: w390 -> [w404 _]
                      tunnel: w389 -> [w411 _]
                      tunnel: w388 -> [w410 w477]
                      tunnel: w379 -> [w409 _]
                      tunnel: w387 -> [w408 w473]
                      tunnel: [w407 w473] -> w386
                      tunnel: [w402 w474] -> w385
                      tunnel: [w406 w471] -> w384
                      tunnel: w382 -> [_ w469]
                      tunnel: w381 -> [w405 w476]
                      tunnel: w379 -> [_ w475]
                      tunnel: w380 -> [w403 w472]
                      frame False {
                        n126 = for {
                          N: w404 -> [w413]
                          tunnel: w410 -> [w428]
                          tunnel: [w418] -> _ mode=indexing
                          tunnel: w405 -> [w429]
                          tunnel: w409 -> [w416]
                          shift-right: [w415] -> w406
                          shift-left: w403 -> [w427]
                          shift-right: [w414] -> w402
                          shift-left: _ -> [_]
                          shift-right: [w421] -> w407
                          shift-left: w408 -> [w421]
                          tunnel: w411 -> [w418]
                          i -> [w420]
                          stop <- w412 stop-if-true
                          n127 = Index Array(array=w427, index=w420) -> (element=w426:T9)
                          n128 = Increment(x=w420) -> (x+1=w419:i32)
                          n129 = Equal?(x=w413, y=w419) -> (x = y?=w417:bool)
                          n130 = Unbundle(w426) -> ("Particle Measurements (Pixels)[0]"=w425:dbl, "Particle Measurements (Pixels)[1]"=w424:dbl)  [unwired: 3 out]
                          n131 = Add(x=w425, y=w418) -> (x+y=w434:dbl)
                          n132 = Subtract(x=w425, y=w418) -> (x-y=w433:dbl)
                          n133 = Add(x=w424, y=w418) -> (x+y=w423:dbl)
                          n134 = Subtract(x=w424, y=w418) -> (x-y=w422:dbl)
                          n135 = In Range and Coerce(upper limit=w434, x=w428, lower limit=w433) -> (In Range?=w432:bool)  [unwired: 1 out]
                          n136 = In Range and Coerce(upper limit=w423, x=w429, lower limit=w422) -> (In Range?=w431:bool)  [unwired: 1 out]
                          n137 = And(x=w432, y=w431) -> (x .and. y?=w430:bool)
                          n138 = case shown="真" w430 {
                            tunnel: w420 -> [w440 w462]
                            tunnel: w428 -> [w439 w468]
                            tunnel: w429 -> [w436 w467]
                            tunnel: w416 -> [w441 w466]
                            tunnel: w427 -> [w443 w465]
                            tunnel: [w442 w464] -> w415
                            tunnel: w421 -> [w438 w461]
                            tunnel: w417 -> [w444 _]
                            tunnel: [w437 w460] -> w414
                            tunnel: w413 -> [_ w460]
                            tunnel: [w435 TRUE] -> w412
                            frame False {
                              n139 = case shown="真" w444 {
                                tunnel: w443 -> [w447 w458]
                                tunnel: [w447 w457] -> w442
                                tunnel: w436 -> [_ w449]
                                tunnel: w439 -> [_ w456]
                                tunnel: w440 -> [w446 w455]
                                tunnel: [w446 w453] -> w437
                                tunnel: w438 -> [_ w452]
                                tunnel: w441 -> [_ w450]
                                tunnel: [FALSE TRUE] -> w435
                                frame False {
                                }
                                frame True {
                                n140 = Add(x=w455, y=1) -> (x+y=w453:i32)
                                n141 = Bundle(w453, "Particle Measurements (Pixels)[0]"=w456, "Particle Measurements (Pixels)[1]"=w449, "Particle Measurements (Pixels)[2]"=w450, w452) -> (w451:T9)  [unwired: 1 out]
                                n142 = Insert Into Array(array=w458, index=w453, new element=w451) -> (w457:T10)
                                }
                              }
                            }
                            frame True {
                              n143 = Bundle(w462, "Particle Measurements (Pixels)[0]"=w468, "Particle Measurements (Pixels)[1]"=w467, "Particle Measurements (Pixels)[2]"=w466, w461) -> (w463:T9)  [unwired: 1 out]
                              n144 = Replace Array Subset(array=w465, new element=w463, index=w462) -> (w464:T10)
                            }
                          }
                        }
                      }
                      frame True {
                        n145 = Bundle(w469, "Particle Measurements (Pixels)[0]"=w477, "Particle Measurements (Pixels)[1]"=w476, "Particle Measurements (Pixels)[2]"=w475, w473) -> (w470:T9)  [unwired: 1 out]
                        n146 = Insert Into Array(array=w472, index=w469, new element=w470) -> (w471:T10)
                      }
                    }
                    n147 = call "IMAQ Overlay Text"("Text Color (black)"=u32 3407634, "Font, Size & Style"=w394, "error in (no error)"=w401, "String"=w398, "Origin"=w395, "Image"=w392) -> ("error out"=w400:errorcluster, "Image Out"=w399:T1)  [unwired: 2 in, 2 out]
                  }
                  n148 = local write "Source Image 5"(w291) -> ()
                  n149 = First Call?() -> (First Call?: T/F=w300:bool)
                  n150 = for {
                    N: w307 -> [_]
                    shift-right: [w360] -> _
                    shift-left: w308 -> [w360]
                    tunnel: w306 -> [w363]
                    tunnel: [w361] -> w305 mode=indexing
                    tunnel: w300 -> [w358]
                    i -> [w369]
                    n151 = Index Array(array=w360, index=w369) -> (element=w368:T9)
                    n152 = Unbundle(w368) -> (w367:i32, "Particle Measurements (Pixels)[0]"=w366:dbl, "Particle Measurements (Pixels)[1]"=w365:dbl, "Particle Measurements (Pixels)[2]"=w364:dbl, w362:i32)
                    n153 = Equal?(x=w362, y=w363) -> (x = y?=w359:bool)
                    n154 = Or(x=w358, y=w359) -> (x .or. y?=w357:bool)
                    n155 = case shown="真" w357 {
                      tunnel: w367 -> [_ w374]
                      tunnel: w366 -> [_ w376]
                      tunnel: w365 -> [_ w375]
                      tunnel: w364 -> [w370 w372]
                      tunnel: w362 -> [_ w373]
                      tunnel: [w370 w372] -> w361
                      frame False {
                      }
                      frame True {
                        n156 = Merge Signals(w373, w374, w376, w375, w372) -> (w377:dynamicdata)
                        n157 = call "创建表格3"("Signals"=w377) -> ("Table"=w371:string[][])  [unwired: 9 in, 1 out]
                        n158 = local read "文件路径输入控件 4"() -> (w378:path)
                        n159 = property on="多列列表框 3" class="MCListbox (严格)"("ItemNames"=w371) -> ()  [unwired: 2 in, 2 out]
                        n160 = call "写入测量文件2"("Signals"=w377, "Filename"=w378) -> ()  [unwired: 15 in, 3 out]
                      }
                    }
                  }
                  n161 = Build Array (concatenate)(w304, w305) -> (w303:dbl[][])
                  n162 = local read "Save\nImage"() -> (w293:bool)
                  n163 = Transpose 2D Array(2D array=w303) -> (transposed array=w316:dbl[][])
                  n164 = Bundle(0, 0.1, w316) -> (w314:cluster{i32, dbl, dbl[][]})  [unwired: 1 out]
                  n165 = case shown="假" w293 {
                    tunnel: w292 -> [w350 w356]
                    tunnel: w291 -> [_ w355]
                    tunnel: w290 -> [w351 w354]
                    tunnel: [w351 w353] -> w289
                    tunnel: [w350 w352] -> w288
                    frame False {
                    }
                    frame True {
                      n166 = call "IMAQ AVI Write Frame"("error in (no error)"=w354, "Image"=w355, "Avi Refnum"=w356) -> ("error out"=w353:errorcluster, "Avi Refnum (duplicate)"=w352:T3)  [unwired: 7 in]
                    }
                  }
                  n167 = local write "数据显示 2"(w314) -> ()
                }
                n168 = VISA Write(VISA resource name=w280, write buffer="ÿý" ("写入缓冲区")) -> (VISA resource name out=w286:refnum<visa-resource-name>, error out=w279:errorcluster)  [unwired: 1 in, 1 out]
                n169 = while {
                  shift-right: [w483] -> _
                  shift-left: dbl[] [] -> [w487]
                  tunnel: w286 -> [w489]
                  tunnel: [w482] -> w282
                  shift-right: [w481] -> w278
                  shift-left: w279 -> [w488]
                  stop <- w480 stop-if-true
                  n170 = VISA Read(VISA resource name=w489, byte count=u32 14 ("字节总数"), error in (no error)=w488) -> (VISA resource name out=w484:refnum<visa-resource-name>, read buffer=w486:string, error out=w485:errorcluster)  [unwired: 1 out]
                  n171 = Unbundle By Name(w485) -> ("status"=w479:bool)
                  n172 = Not(x=w479) -> (.not. x?=w478:bool)
                  n173 = case shown="真" w478 {
                    tunnel: w487 -> [w501 w516]
                    tunnel: w486 -> [_ w515]
                    tunnel: w485 -> [w499 w527]
                    tunnel: w484 -> [w496 w528]
                    tunnel: [w501 w529] -> w483
                    tunnel: [w497 w528] -> w482
                    tunnel: [w491 w527] -> w481
                    tunnel: [FALSE w526] -> w480
                    frame False {
                      n174 = call <vilib>:"Clear Errors.vi"("error in (no error)"=w499) -> ()  [unwired: 7 out]
                      n175 = VISA Clear(VISA resource name=w496) -> (VISA resource name out=w493:refnum<visa-resource-name>, error out=w495:errorcluster)  [unwired: 1 in]
                      n176 = call <vilib>:"Clear Errors.vi"("error in (no error)"=w495) -> ("error out"=w494:errorcluster)  [unwired: 6 out]
                      n177 = VISA Write(VISA resource name=w493, write buffer="ÿð" ("写入缓冲区"), error in (no error)=w494) -> (VISA resource name out=w497:refnum<visa-resource-name>, error out=w492:errorcluster)  [unwired: 1 out]
                      n178 = call <vilib>:"Clear Errors.vi"("error in (no error)"=w492) -> ("error out"=w491:errorcluster)  [unwired: 6 out]
                    }
                    frame True {
                      w531 = 0  # x0
                      # "motor_d"
                      # "motor_c"
                      # "motor_a"
                      # "time"
                      # "motor_d"
                      # "temp"
                      # "簇作为输入时需要指定3个元素：\n起始位置x0，数据点间隔dx，数组数据"
                      n179 = String Subset ("截取字符串6")(string=w515, offset (0)=6, length (rest)=1 ("长度（剩余）")) -> (substring=w557:string)
                      n180 = Bundle("x0"=w531, "y"=0.1, w516) -> (→"数据显示":cluster{"x0":i32, "y":dbl, dbl[]})  [unwired: 1 out]
                      n181 = String Subset ("截取字符串4")(string=w515, offset (0)=4, length (rest)=1 ("长度（剩余）")) -> (substring=w556:string)
                      n182 = String Subset ("截取字符串5")(string=w515, offset (0)=5, length (rest)=1 ("长度（剩余）")) -> (substring=w586:string)
                      n183 = String Subset ("截取字符串7")(string=w515, offset (0)=7, length (rest)=1 ("长度（剩余）")) -> (substring=w592:string)
                      n184 = String Subset ("截取字符串8")(string=w515, offset (0)=8, length (rest)=1 ("长度（剩余）")) -> (substring=w558:string)
                      n185 = String Subset ("截取字符串9")(string=w515, offset (0)=9, length (rest)=1 ("长度（剩余）")) -> (substring=w597:string)
                      n186 = String Subset ("截取字符串2")(string=w515, offset (0)=2, length (rest)=1 ("长度（剩余）")) -> (substring=w542:string)
                      n187 = String Subset ("截取字符串3")(string=w515, offset (0)=3, length (rest)=1 ("长度（剩余）")) -> (substring=w555:string)
                      n188 = String Subset ("截取字符串10")(string=w515, offset (0)=10, length (rest)=1 ("长度（剩余）")) -> (substring=w559:string)
                      n189 = String Subset ("截取字符串11")(string=w515, offset (0)=11, length (rest)=1 ("长度（剩余）")) -> (substring=w603:string)
                      n190 = String Subset ("截取字符串11")(string=w515, offset (0)=12) -> (substring=w511:string)  [unwired: 1 in]
                      n191 = String Subset ("截取字符串11")(string=w515, offset (0)=13) -> (substring=w512:string)  [unwired: 1 in]
                      n192 = call "Convert Hex String to ASCII Hex.vi"("“十六进制显示”字符串"=w556) -> ("“正常显示”字符串"=w587:string)  [unwired: 2 in]
                      n193 = call "Convert Hex String to ASCII Hex.vi"("“十六进制显示”字符串"=w597) -> ("“正常显示”字符串"=w599:string)  [unwired: 2 in]
                      n194 = call "Convert Hex String to ASCII Hex.vi"("“十六进制显示”字符串"=w555) -> ("“正常显示”字符串"=w562:string)  [unwired: 2 in]
                      n195 = call "Convert Hex String to ASCII Hex.vi"("“十六进制显示”字符串"=w557) -> ("“正常显示”字符串"=w594:string)  [unwired: 2 in]
                      n196 = call "Convert Hex String to ASCII Hex.vi"("“十六进制显示”字符串"=w586) -> ("“正常显示”字符串"=w588:string)  [unwired: 2 in]
                      n197 = call "Convert Hex String to ASCII Hex.vi"("“十六进制显示”字符串"=w592) -> ("“正常显示”字符串"=w593:string)  [unwired: 2 in]
                      n198 = call "Convert Hex String to ASCII Hex.vi"("“十六进制显示”字符串"=w558) -> ("“正常显示”字符串"=w600:string)  [unwired: 2 in]
                      n199 = call "Convert Hex String to ASCII Hex.vi"("“十六进制显示”字符串"=w542) -> ("“正常显示”字符串"=w563:string)  [unwired: 2 in]
                      n200 = Concatenate Strings "连接字符串"(w587, w588) -> (w589:string)
                      n201 = Concatenate Strings "连接字符串"(w594, w593) -> (w595:string)
                      n202 = Concatenate Strings "连接字符串"(w600, w599) -> (w601:string)
                      n203 = call "Convert Hex String to ASCII Hex.vi"("“十六进制显示”字符串"=w603) -> ("“正常显示”字符串"=w606:string)  [unwired: 2 in]
                      n204 = Concatenate Strings "连接字符串"(w563, w562) -> (w582:string)
                      n205 = call "Convert Hex String to ASCII Hex.vi"("“十六进制显示”字符串"=w559) -> ("“正常显示”字符串"=w605:string)  [unwired: 2 in]
                      n206 = call "Convert Hex String to ASCII Hex.vi"("“十六进制显示”字符串"=w511) -> ("“正常显示”字符串"=w510:string)  [unwired: 2 in]
                      n207 = call "Convert Hex String to ASCII Hex.vi"("“十六进制显示”字符串"=w512) -> ("“正常显示”字符串"=w509:string)  [unwired: 2 in]
                      n208 = Concatenate Strings "连接字符串"(w605, w606) -> (w607:string)
                      n209 = Concatenate Strings "连接字符串"(w510, w509) -> (w506:string)
                      n210 = Hexadecimal String To Number "motor_a"(string=w589) -> (number=w577:u32)  [unwired: 1 in, 2 out]
                      "Injector 1" <- w577
                      n211 = Hexadecimal String To Number "motor_b"(string=w595) -> (number=w578:u32)  [unwired: 3 out]
                      "Injector 2" <- w578
                      n212 = Hexadecimal String To Number "motor_c"(string=w601) -> (number=w579:u32)  [unwired: 3 out]
                      "Injector 3" <- w579
                      n213 = Hexadecimal String To Number "temp"(string=w582) -> (number=w575:u32)  [unwired: 3 out]
                      n214 = Hexadecimal String To Number "motor_d"(string=w607) -> (number=w580:u32)  [unwired: 3 out]
                      "Refrigerator" <- w580
                      n215 = Hexadecimal String To Number "motor_d"(string=w506) -> (number=w505:u32)  [unwired: 3 out]
                      "Heater" <- w505
                      n216 = To Double Precision Float(number=w575) -> (double precision float=w543:dbl)
                      n217 = String Subset "截取字符串0"(string=w515, offset (0)=0 ("偏移量(0)"), length (rest)=1 ("length (rest)")) -> (substring=w540:string)
                      n218 = String Subset "截取字符串1"(string=w515, offset (0)=1, length (rest)=1 ("长度（剩余）")) -> (substring=w541:string)
                      n219 = Multiply(x=1.0, y=w543) -> (x*y=w565:dbl)
                      n220 = Subtract(x=w565, y=500.0 ("x")) -> (x-y=w503:dbl)
                      "tmp" <- w503
                      "数值显示控件" <- w503
                      n221 = Array Size "数组大小"(array=w516) -> (size(s)=w530:i32)
                      n222 = call "Convert Hex String to ASCII Hex.vi"("“十六进制显示”字符串"=w540) -> ("“正常显示”字符串"=w560:string)  [unwired: 2 in]
                      n223 = call "Convert Hex String to ASCII Hex.vi"("“十六进制显示”字符串"=w541) -> ("“正常显示”字符串"=w561:string)  [unwired: 2 in]
                      n224 = Concatenate Strings "连接字符串"(w560, w561) -> (w581:string)
                      n225 = Insert Into Array "数组插入"(array=w516, index=w530, new element=w503) -> (w529:dbl[])
                      n226 = Hexadecimal String To Number "time"(string=w581) -> (number=w576:u32)  [unwired: 3 out]
                      n227 = To Double Precision Float(number=w577) -> (double precision float=w567:dbl)
                      n228 = To Double Precision Float(number=w578) -> (double precision float=w573:dbl)
                      n229 = To Double Precision Float(number=w579) -> (double precision float=w571:dbl)
                      n230 = To Double Precision Float(number=w580) -> (double precision float=w569:dbl)
                      n231 = To Double Precision Float(number=w505) -> (double precision float=w507:dbl)
                      n232 = To Double Precision Float(number=w576) -> (double precision float=w583:dbl)
                      n233 = Multiply(x=0.01, y=w567) -> (x*y=w525:dbl)
                      "数值 1" <- w525
                      n234 = Multiply(x=0.01, y=w573) -> (x*y=w524:dbl)
                      "数值 2" <- w524
                      n235 = Multiply(x=0.01, y=w571) -> (x*y=w523:dbl)
                      "数值 3" <- w523
                      n236 = Multiply(x=0.01, y=w569) -> (x*y=w522:dbl)
                      "数值 4" <- w522
                      n237 = Multiply(x=0.01, y=w507) -> (x*y=w504:dbl)
                      "数值 5" <- w504
                      n238 = Multiply(x=0.01, y=w583) -> (x*y=w521:dbl)
                      n239 = Merge Signals(w521, w503, w525, w524, w523, w522, w504) -> (w518:dynamicdata)
                      n240 = call "写入测量文件"("Signals"=w518, "Filename"="文件路径输入控件") -> ()  [unwired: 15 in, 3 out]
                      n241 = call "创建表格"("Signals"=w518) -> ("Table"=w520:string[][])  [unwired: 9 in, 1 out]
                      n242 = local read "停止采集"() -> (w502:bool)
                      n243 = local read "退出"() -> (w544:bool)
                      n244 = property on="多列列表框" class="MCListbox (严格)"("ItemNames"=w520) -> ()  [unwired: 2 in, 2 out]
                      n245 = Or(x=w544, y=w502) -> (x .or. y?=w526:bool)
                    }
                  }
                }
                n246 = VISA Write(VISA resource name=w282, write buffer="ÿÿ" ("写入缓冲区"), error in (no error)=w278) -> (VISA resource name out=w284:refnum<visa-resource-name>, error out=w283:errorcluster)  [unwired: 1 out]
                n247 = VISA Close "VISA关闭"(VISA resource name=w284, error in (no error)=w283) -> (error out=w281:errorcluster)
                n248 = call <vilib>:"Clear Errors.vi"("error in (no error)"=w281) -> ()  [unwired: 7 out]
              }
            }
          }
          event "建立过程": Value Change {
            # "自动识别开发板所连接的串口"
            n249 = event-data() -> ()  [unwired: 6 out]
            n250 = call "find com.vi"() -> ("连接了开发板？"=w612:bool, "VISA resource name out"=w613:refnum<visa-resource-name>)  [unwired: 2 in]
            n251 = case shown="真" w612 {
              tunnel: w613 -> [_ w619]
              frame False {
                n252 = One Button Dialog(message="没有找到外设。请检查电源、连接，以及程序。" ("消息"), button name ("OK")="确定" ("按钮名称（“确定”）")) -> ()  [unwired: 1 out]
              }
              frame True {
                # "发送0xff给STM32。STM32收到0xff之后，\n发现不是0xf0，那么就停止数据采集"
                # "发送0xf1给STM32。\nSTM32收到0xf1之后，\n开始建立过程"
                n253 = VISA Write(VISA resource name=w619, write buffer="ÿþ" ("写入缓冲区")) -> (VISA resource name out=w618:refnum<visa-resource-name>)  [unwired: 1 in, 2 out]
                n254 = while {
                  tunnel: w618 -> [w640]
                  shift-right: [w629] -> w617
                  shift-left: _ -> [_]
                  tunnel: [w628] -> w616
                  stop <- w631 stop-if-true
                  # "x"
                  # "Y"
                  n255 = property on="多列列表框 2" class="MCListbox (严格)"() -> ("ItemNames"=w635:string[][])  [unwired: 2 in, 2 out]
                  n256 = Array Size(array=w635) -> (size(s)=w634:i32[])
                  n257 = Transpose 2D Array(2D array=w635) -> (transposed array=w636:string[][])
                  n258 = Array Size(array=w636) -> (size(s)=w638:i32[])
                  n259 = Index Array(array=w634, index=0) -> (element=w633:i32)
                  n260 = Index Array(array=w638, index=0) -> (element=w632:i32)
                  n261 = for "For循环" {
                    N: w633 -> [w644]
                    tunnel: w640 -> [w648]
                    tunnel: w632 -> [w645]
                    tunnel: [w647] -> _ mode=indexing
                    tunnel: [w643] -> _ mode=indexing
                    shift-right: [w642] -> w629
                    shift-left: _ -> [_]
                    shift-right: [w641] -> w628
                    shift-left: _ -> [_]
                    i -> [w646]
                    # "y"
                    n262 = for "For循环" {
                      N: w645 -> [w664]
                      tunnel: w648 -> [w670]
                      tunnel: [w649] -> w647 mode=indexing
                      tunnel: w646 -> [w661]
                      tunnel: w644 -> [w669]
                      tunnel: [w651] -> w643 mode=indexing
                      shift-right: [w651] -> w642
                      shift-left: _ -> [_]
                      shift-right: [w649] -> w641
                      shift-left: _ -> [_]
                      i -> [w662]
                      # "x"
                      n263 = property on="多列列表框 2" class="MCListbox (严格)"() -> ("ItemNames"=w666:string[][])  [unwired: 2 in, 2 out]
                      n264 = Transpose 2D Array(2D array=w666) -> (transposed array=w665:string[][])
                      n265 = Index Array(array=w665, index (row)=w662, index (col)=w661) -> (element=w659:string)
                      n266 = Hexadecimal String To Number(string=w659) -> (number=w657:u32)  [unwired: 2 in, 1 out]
                      n267 = Split Number(x=w657) -> (lo(x)=w656:u16)  [unwired: 1 out]
                      n268 = Wait (ms)(milliseconds to wait=0) -> ()  [unwired: 1 out]
                      n269 = Split Number(x=w656) -> (hi(x)=w653:u8, lo(x)=w655:u8)
                      n270 = Increment(x=w662) -> (x+1=w663:i32)
                      n271 = Increment(x=w661) -> (x+1=w660:i32)
                      n272 = Type Cast(x=w653) -> (*(type *) &x=w652:string)  [unwired: 1 in]
                      n273 = Equal?(x=w664, y=w663) -> (x = y?=w668:bool)
                      n274 = Equal?(x=w660, y=w669) -> (x = y?=w667:bool)
                      n275 = VISA Write(VISA resource name=w670, write buffer=w652) -> (VISA resource name out=w658:refnum<visa-resource-name>)  [unwired: 1 in, 2 out]
                      n276 = Type Cast(x=w655) -> (*(type *) &x=w654:string)  [unwired: 1 in]
                      n277 = VISA Write(VISA resource name=w658, write buffer=w654) -> (VISA resource name out=w649:refnum<visa-resource-name>)  [unwired: 1 in, 2 out]
                      n278 = And(x=w668, y=w667) -> (x .and. y?=w651:bool)
                    }
                  }
                  n279 = local read "退出"() -> (w630:bool)
                  n280 = Or(x=w630, y=w629) -> (x .or. y?=w631:bool)
                }
                n281 = case shown="真" w617 {
                  tunnel: w616 -> [_ w621]
                  frame False {
                  }
                  frame True {
                    # "释放串口"
                    n282 = VISA Write(VISA resource name=w621, write buffer="ÿÿ" ("写入缓冲区")) -> (VISA resource name out=w623:refnum<visa-resource-name>, error out=w624:errorcluster)  [unwired: 1 in, 1 out]
                    n283 = VISA Close "VISA关闭"(VISA resource name=w623, error in (no error)=w624) -> (error out=w625:errorcluster)
                    n284 = One Button Dialog(message="过程已建立成功" ("消息"), button name ("OK")="确定" ("按钮名称（“确定”）")) -> ()  [unwired: 1 out]
                    n285 = call <vilib>:"Clear Errors.vi"("error in (no error)"=w625) -> ()  [unwired: 7 out]
                  }
                }
              }
            }
            n286 = call-poly <vilib>:"Read From Spreadsheet File.vi"("file path (dialog if empty)"="文件路径输入控件 2") -> ("all rows"=w609:dbl[][])  [unwired: 6 in, 4 out]
            n287 = Number To Hexadecimal String(2:w609) -> (0:w608:string[][])  [unwired: 1 in]
            n288 = property on="多列列表框 2" class="MCListbox (严格)"("ItemNames"=w608) -> ()  [unwired: 2 in, 2 out]
          }
          event "退出": Value Change {
            n289 = event-data() -> ()  [unwired: 7 out]
          }
          event "搜索按钮": Value Change {
            n290 = event-data() -> ()  [unwired: 7 out]
            n291 = while {
              tunnel: [w692] -> w676
              tunnel: w675 -> [w686]
              tunnel: w674 -> [w685]
              tunnel: w673 -> [w684]
              stop <- w678 stop-if-true
              w699 = T4[] [0, 3, 35] items=["Center of Mass X", "Center of Mass Y", "First Pixel X", "First Pixel Y", "Bounding Rect Left", "Bounding Rect Top", "Bounding Rect Right", "Bounding Rect Bottom", "Max Feret Diameter Start X", "Max Feret Diameter Start Y", "Max Feret Diameter End X", "Max Feret Diameter End Y", "Max Horiz. Segment Length Left", "Max Horiz. Segment Length Right", "Max Horiz. Segment Length Row", "-", "Bounding Rect Width", "Bounding Rect Height", "Bounding Rect Diagonal", "Perimeter", "Convex Hull Perimeter", "Holes' Perimeter", "Max Feret Diameter", "Equivalent Ellipse Major Axis", "Equivalent Ellipse Minor Axis", "Equivalent Ellipse Minor Axis (Feret)", "Equivalent Rect Long Side", "Equivalent Rect Short Side", "Equivalent Rect Diagonal", "Equivalent Rect Short Side (Feret)", "Average Horiz. Segment Length", "Average Vert. Segment Length", "Hydraulic Radius", "Waddel Disk Diameter", "-", "Area", "Holes' Area", "Particle & Holes' Area", "Convex Hull Area", "Image Area", "-", "Number of Holes", "Number of Horiz. Segments", "Number of Vert. Segments", "-", "Orientation", "Max Feret Diameter Orientation", "-", "% Area/Image Area", "% Area/(Particle & Holes' Area)", "Ratio of Equivalent Ellipse Axes", "Ratio of Equivalent Rect Sides", "-", "Elongation Factor", "Compactness Factor", "Heywood Circularity Factor", "Type Factor", "-", "Sum X", "Sum Y", "Sum XX", "Sum XY", "Sum YY", "Sum XXX", "Sum XXY", "Sum XYY", "Sum YYY", "-", "Moment of Inertia XX", "Moment of Inertia XY", "Moment of Inertia YY", "Moment of Inertia XXX", "Moment of Inertia XXY", "Moment of Inertia XYY", "Moment of Inertia YYY", "Norm. Moment of Inertia XX", "Norm. Moment of Inertia XY", "Norm. Moment of Inertia YY", "Norm. Moment of Inertia XXX", "Norm. Moment of Inertia XXY", "Norm. Moment of Inertia XYY", "Norm. Moment of Inertia YYY", "Hu Moment 1", "Hu Moment 2", "Hu Moment 3", "Hu Moment 4", "Hu Moment 5", "Hu Moment 6", "Hu Moment 7"] ("Pixel Measurements")
              n292 = call <vilib>:"IMAQdx Grab.vi"("error in"=w686, "Image In"=w685, "Session In"=w684) -> ("error out"=w716:errorcluster, "Image Out"=w714:T1)  [unwired: 5 in, 2 out]
              n293 = Wait (ms)(milliseconds to wait=100 ("Kernel Number")) -> ()  [unwired: 1 out]
              n294 = local read "停止按钮"() -> (w679:bool)
              n295 = call "IMAQ Cast Image"("error in (no error)"=w716, "Image Src"=w714) -> ("error out"=w715:errorcluster, "Image Dst Out"=w691:T1)  [unwired: 8 in]
              n296 = local read "退出"() -> (w680:bool)
              n297 = local write "Source Image"(w691) -> ()
              n298 = call "IMAQ Inverse"("error in (no error)"=w715, "Image Src"=w691) -> ("error out"=w713:errorcluster, "Image Dst Out"=w690:T1)  [unwired: 8 in]
              n299 = local write "Source Image 2"(w690) -> ()
              n300 = Or(x=w680, y=w679) -> (x .or. y?=w678:bool)
              n301 = call "IMAQ GetKernel"("error in (no error)"=w713, "Kernel Number"=5, "Kernel Size (3,5,...)"=3) -> ("error out"=w712:errorcluster, "Kernel"=w683:sgl[][])  [unwired: 2 in, 5 out]
              n302 = call "IMAQ Convolute"("Kernel"=w683, "error in (no error)"=w712, "Image Src"=w690) -> ("error out"=w711:errorcluster, "Image Dst Out"=w704:T1)  [unwired: 4 in, 3 out]
              n303 = call "IMAQ Threshold"("error in (no error)"=w711, "Range"="Threshold Value", "Image Src"=w704) -> ("error out"=w710:errorcluster, "Image Dst Out"=w689:T1)  [unwired: 3 in, 4 out]
              n304 = local write "Source Image 3"(w689) -> ()
              n305 = call "IMAQ FillHole"("error in (no error)"=w710, "Image Src"=w689) -> ("error out"=w709:errorcluster, "Image Dst Out"=w703:T1)  [unwired: 2 in, 2 out]
              n306 = call "IMAQ RejectBorder"("error in (no error)"=w709, "Image Src"=w703) -> ("error out"=w708:errorcluster, "Image Dst Out"=w702:T1)  [unwired: 2 in, 2 out]
              n307 = call "IMAQ RemoveParticle"("error in (no error)"=w708, "Number of Erosion"=5 ("Kernel Number"), "Image Src"=w702) -> ("error out"=w700:errorcluster, "Image Dst Out"=w688:T1)  [unwired: 4 in, 3 out]
              n308 = local read "Font, Size & Style"() -> (w696:T2)
              n309 = local write "Source Image 4"(w688) -> ()
              n310 = call "IMAQ Particle Filter 3"("Image Src"=w688, "Selection Values"=T5 [{"Measurement Parameter"=55, "Range Lower Value"=0.0, "Range Upper Value"=1.06, "Range"=FALSE, "Measurement Type"=FALSE}], "error in (no error)"=w700) -> ("Image Dst Out"=w697:T1, "error out"=w698:errorcluster)  [unwired: 6 in, 5 out]
              n311 = call "IMAQ Particle Analysis"("error in (no error)"=w698, "Pixel Measurements"=w699, "Image"=w697) -> ("error out"=w694:errorcluster, "Particle Measurements (Pixels)"=w695:dbl[][], "Image Out (duplicate)"=w693:T1)  [unwired: 2 in, 4 out]
              n312 = for "For循环" {
                tunnel: [w717] -> _ mode=indexing
                tunnel: [w729] -> w692
                tunnel: [w728] -> w687
                tunnel: w696 -> [w722]
                tunnel: w695 -> [w721] mode=indexing
                tunnel: w693 -> [w720]
                tunnel: [w718] -> _ mode=indexing
                tunnel: w694 -> [w717]
                n313 = Array To Cluster(array=w721) -> (cluster=w725:T7)
                n314 = Unbundle(w725) -> ("Particle Measurements (Pixels)[0]"=w719:dbl, "Particle Measurements (Pixels)[1]"=w724:dbl, "Particle Measurements (Pixels)[2]"=w718:dbl)
                n315 = Bundle("Particle Measurements (Pixels)[0]"=w719, "Particle Measurements (Pixels)[1]"=w724) -> (w723:T8)  [unwired: 1 out]
                n316 = Number To Decimal String(number=w718) -> (decimal integer string=w727:string)  [unwired: 1 out]
                n317 = call "IMAQ Overlay Text"("Text Color (black)"=u32 3407634, "Font, Size & Style"=w722, "error in (no error)"=w717, "String"=w727, "Origin"=w723, "Image"=w720) -> ("error out"=w729:errorcluster, "Image Out"=w728:T1)  [unwired: 2 in, 2 out]
              }
              n318 = local write "Source Image 5"(w687) -> ()
            }
            n319 = call "IMAQ Dispose"("error in (no error)"=w676) -> ("error out"=w677:errorcluster)  [unwired: 5 in]
            n320 = call <vilib>:"Clear Errors.vi"("error in (no error)"=w677) -> ()  [unwired: 7 out]
          }
          event Timeout {
            n321 = event-data() -> ()  [unwired: 4 out]
          }
        }
      }
    }
  }
  n322 = call "IMAQ Dispose"("error in (no error)"=w11) -> ("error out"=w15:errorcluster)  [unwired: 5 in]
  n323 = call <vilib>:"IMAQdx Close Camera.vi"("error in"=w3, "Session In"=w2) -> ("error out"=w16:errorcluster)  [unwired: 9 in]
  n324 = call "IMAQ AVI Close"("error in (no error)"=w12, "Avi Refnum"=w14) -> ("error out"=w13:errorcluster)  [unwired: 9 in]
  n325 = call <vilib>:"Clear Errors.vi"("error in (no error)"=w15) -> ()  [unwired: 7 out]
  n326 = call <vilib>:"Clear Errors.vi"("error in (no error)"=w16) -> ()  [unwired: 7 out]
  n327 = call <vilib>:"Clear Errors.vi"("error in (no error)"=w13) -> ()  [unwired: 7 out]
